vi "rtd daqmx scale type.vi"() -> ()   [LabVIEW 2019]
uses:
  <vilib>/DAQmx/create/channels.llb/DAQmx Create Channel (AI-Temperature-RTD).vi
  <vilib>/DAQmx/configure/timing.llb/DAQmx Timing (Sample Clock).vi
  <vilib>/DAQmx/configure/task.llb/DAQmx Configure Logging (TDMS).vi
panel:
  out "Error Out":errorcluster
  in  "TDMS File":path=path "C:/Python/projects/nitdms/tests/tdms_files/rtd daqmx scale type.tdms"
  in  "DAQmx Physical Channel":tag="cDAQ1Mod1/ai0"
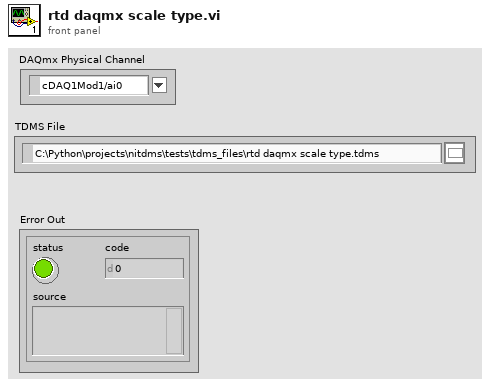
[diagram p1: front panel]
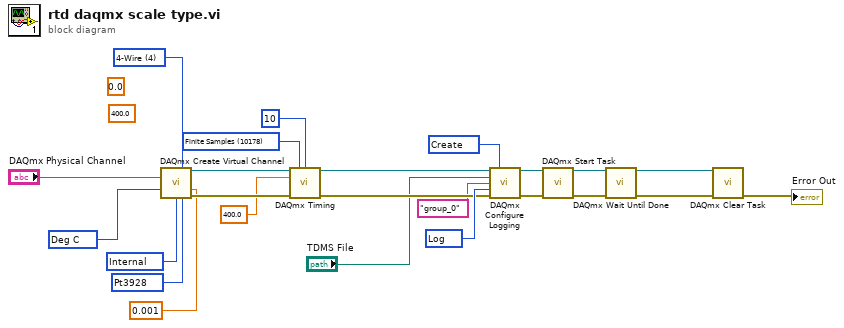
[diagram p0: block diagram]
diagram:
  w2 = 10200 items=["Internal"=10200, "External"=10167, "None"=10230] ("current excitation source")
  w3 = 12483 items=["Pt3750"=12481, "Pt3851"=10071, "Pt3911"=12482, "Pt3916"=10069, "Pt3920"=10053, "Pt3928"=12483, "Custom"=10137] ("rtd type")
  w4 = 4 items=["2-Wire"=2, "3-Wire"=3, "4-Wire"=4] ("resistance configuration")
  w5 = 10143 items=["Deg C"=10143, "Deg F"=10144, "Kelvins"=10325, "Deg R"=10145, "From Custom Scale"=10065] ("units")
  (unwired) 0.0
  w19 = 10178 items=["Finite Samples"=10178, "Continuous Samples"=10123, "Hardware Timed Single Point"=12522] ("sample mode")
  w22 = 15848 items=["Open"=10437, "Open or Create"=15846, "Create or Replace"=15847, "Create"=15848] ("operation")
  w23 = 15844 items=["Off"=10231, "Log"=15844, "Log and Read"=15842] ("logging mode")
  (unwired) 400.0
  n1 = call-poly <vilib>:"DAQmx Create Virtual Channel.vi"("resistance configuration"=w4, "physical channels"="DAQmx Physical Channel", "units"=w5, "current excitation value"=0.001, "current excitation source"=w2, "rtd type"=w3) -> ("task out"=w20:refnum<k21>, "error out"=w21:errorcluster)  [unwired: 8 in]
  n2 = call-poly <vilib>:"DAQmx Timing.vi"("task/channels in"=w20, "sample mode"=w19, "samples per channel"=10, "rate"=400.0, "error in"=w21) -> ("task out"=w15:refnum<k21>, "error out"=w16:errorcluster)  [unwired: 9 in]
  n3 = call-poly <vilib>:"DAQmx Configure Logging.vi"("task/channels in"=w15, "operation"=w22, "file path"="TDMS File", "group name"="group_0", "logging mode"=w23, "error in"=w16) -> ("task out"=w10:refnum<k21>, "error out"=w11:errorcluster)  [unwired: 8 in]
  n4 = call <vilib>:"DAQmx Start Task.vi"("task/channels in"=w10, "error in"=w11) -> ("task out"=w8:refnum<k21>, "error out"=w9:errorcluster)  [unwired: 12 in]
  n5 = call <vilib>:"DAQmx Wait Until Done.vi"("task/channels in"=w8, "error in"=w9) -> ("task out"=w6:refnum<k21>, "error out"=w7:errorcluster)  [unwired: 12 in]
  n6 = call <vilib>:"DAQmx Clear Task.vi"("task in"=w6, "error in"=w7) -> ("error out"=→"Error Out":errorcluster)  [unwired: 13 in]
